vi "op2-Video-AQ.vi"() -> ()   [LabVIEW 2024]
uses:
  <vilib>/userDefined/High Color/IMAQdx.ctl
  <vilib>/vision/driver/NI_Vision_Acquisition_Software.lvlib
panel:
  out "Image":T1(plugin-control)
  in  "Session In":T2
  in  "stop":bool
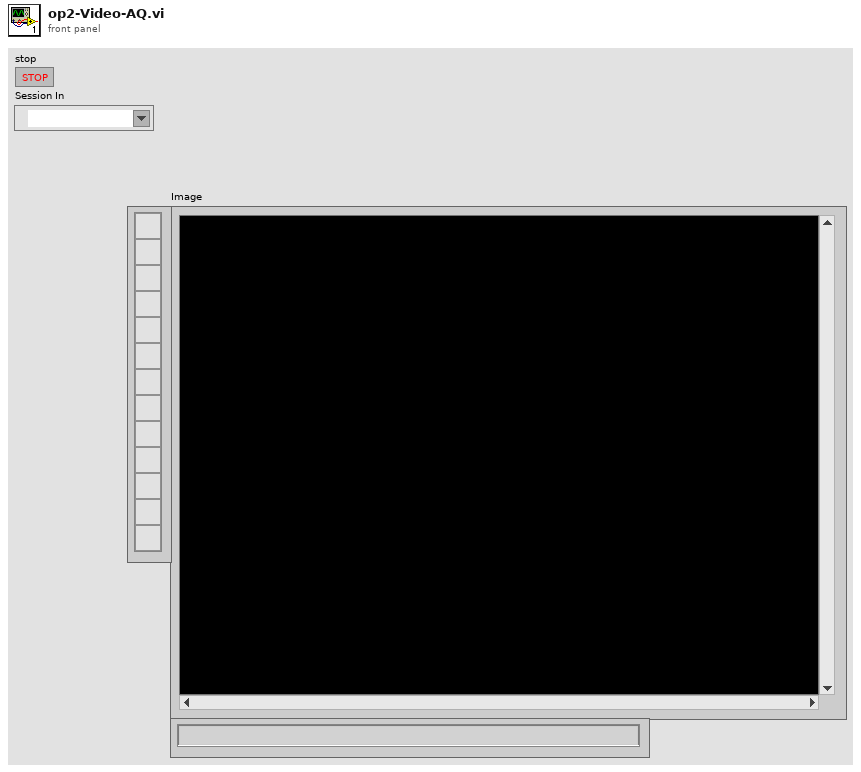
[diagram p1: front panel]
types:
  T1 = typedef "IMAQ Image.ctl" = refnum<image>
  T2 = typedef "IMAQdx.ctl" = refnum<k21>
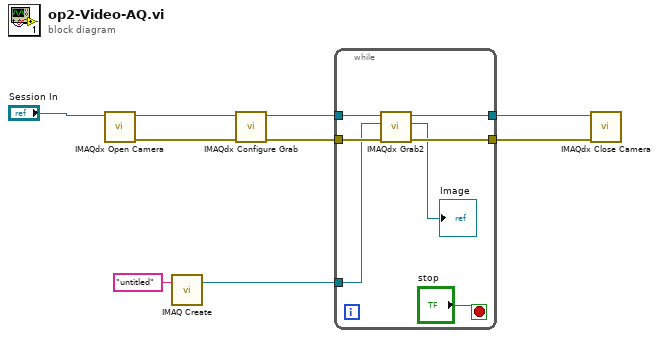
[diagram p0: block diagram]
diagram:
  n1 = call <vilib>:"IMAQdx Open Camera.vi"("Session In"="Session In") -> ("error out"=w6:errorcluster, "Session Out"=w8:T2)  [unwired: 9 in]
  n2 = call "IMAQ Create"("Image Name"="untitled") -> ("New Image"=w2:T1)  [unwired: 4 in, 1 out]
  n3 = call <vilib>:"IMAQdx Configure Grab.vi"("error in"=w6, "Session In"=w8) -> ("error out"=w5:errorcluster, "Session Out"=w7:T2)  [unwired: 8 in]
  n4 = while {
    tunnel: w7 -> [w15]
    tunnel: w5 -> [w14]
    tunnel: [w13] -> w4
    tunnel: [w12] -> w3
    tunnel: w2 -> [w11]
    stop <- "stop" stop-if-true
    n5 = call <vilib>:"IMAQdx Grab2.vi"("error in"=w14, "Image In"=w11, "Session In"=w15) -> ("error out"=w12:errorcluster, "Image Out"=→"Image":T1, "Session Out"=w13:T2)  [unwired: 5 in, 1 out]
  }
  n6 = call <vilib>:"IMAQdx Close Camera.vi"("error in"=w3, "Session In"=w4) -> ()  [unwired: 9 in, 1 out]
